vi "SVFA Get Spectrum Value (NxM).vi"(0 "spectra":T8(array[cluster]) {"magnitude" format="%.2f"; "dx" format="%.2f"; "x0" format="%.2f"}, 2 "x value (1000)":dbl=1000.0 format="%.2f", 3 "coercion (nearest)":T1(ring), 4 "spectrum info":T2[][](array[typedef]) {"x-axis units" items=["Frequency-Arbitrary (Hz)"=0, "Frequency-CB (Hz)"=1, "Frequency-CPB (Hz)"=1248, "Frequency-Arbitrary (Hz)"=2357, "Quefrency (s)"=2, "Revolutions (rev)"=3, "Order"=4, "Speed (RPM)"=11, "Speed (rad/s)"=21, "Index"=65535]; "weighting filter" items=["Linear", "A-weighting", "B-weighting", "C-weighting", "ITU-R 468-4", "Dolby", "CCITT", "C-message", "Wb", "Wc", "Wd", "We", "Wf", "Wh", "Wj", "Wk", "Wm", "AES17 20 kHz lowpass", "AES17 40 kHz lowpass", "AES17 20 kHz highpass", "AES17 40 kHz highpass"]; "dB reference [EU]" format="%.2f"; "engineering units" items=["custom..."=0, "V"=1, "A"=21, "C"=30, "pC"=31, "s"=32, "-"=29, "Pa"=2, "N"=20, "g"=3, "m/s^2"=4, "m/s"=5, "m"=6, "mm/s"=12, "mm"=13, "micron/s"=14, "micron"=15, "in/s^2"=7, "in/s"=8, "in"=9, "mil/s"=10, "mil"=11, "rad/s^2"=16, "rad/s"=17, "rad"=18, "deg/s^2"=26, "deg/s"=27, "deg"=28, "RPM"=22, "cycle/s^2"=23, "Hz"=24, "cycle"=25, "strain"=19]; "spectral info"."window" items=["None "=0, "Hanning"=1, "Hamming"=2, "Blackman-Harris"=3, "Exact Blackman"=4, "Blackman"=5, "Flat Top"=6, "4 Term B-Harris "=7, "7 Term B-Harris"=8, "Low Sidelobe"=9, "Force - Exponential"=10, "Gaussian"=62]}, 5 "error in (no error)":errorcluster) -> (14 "spectra values":dbl[][](array[numeric]), 15 "unit labels":string[][](array[string]), 16 "actual x values":dbl[][](array[numeric]), 17 "x labels":string[][](array[string]), 19 "error out":errorcluster)   [LabVIEW 2017]
doc: "Extracts the value of the spectrum at the specified frequency. Use the frequency coercion control to specify how the frequency should be coerced if it does not exactly coincide with a frequency line. This VI operates on any real-valued spectrum. Wire data to the <B>spectrum</B> input to determine the polymorphic instance to use or manually select the instance."
uses:
  <vilib>/addons/_NISVFA/_Shared subVIs/Controls/svc_Spectrum Info.ctl
  <vilib>/addons/_NISVFA/_Shared subVIs/Controls/svc_X-Axis Units.ctl
  <vilib>/addons/_NISVFA/_Shared subVIs/Controls/svc_Spectrum Type.ctl
  <vilib>/addons/_NISVFA/_Shared subVIs/Controls/svc_Engineering Units Text Ring.ctl
  <vilib>/addons/_NISVFA/_Shared subVIs/Controls/svc_Weighting Filter Text Ring.ctl
  <vilib>/addons/_NISVFA/_Shared subVIs/Controls/svc_Complimentary Spectrum Units.ctl
  <vilib>/addons/_NISVFA/_Shared subVIs/Common/svc_Spectrum Units.vi
  <vilib>/addons/_NISVFA/_Shared subVIs/Common/svc_Convert Frequency to Frequency String.vi
  <vilib>/addons/_NISVFA/_Shared subVIs/Common/svc_Get Weighting Enum and Labels.vi
  <vilib>/addons/_NISVFA/_Shared subVIs/Common/svc_Unit Label Lexical Class.vi
  <vilib>/addons/_NISVFA/_Shared subVIs/Common/svc_Engineering Units to Unit Label.vi
  <vilib>/addons/_NISVFA/_Shared subVIs/Common/svc_Format Value (DBL).vi
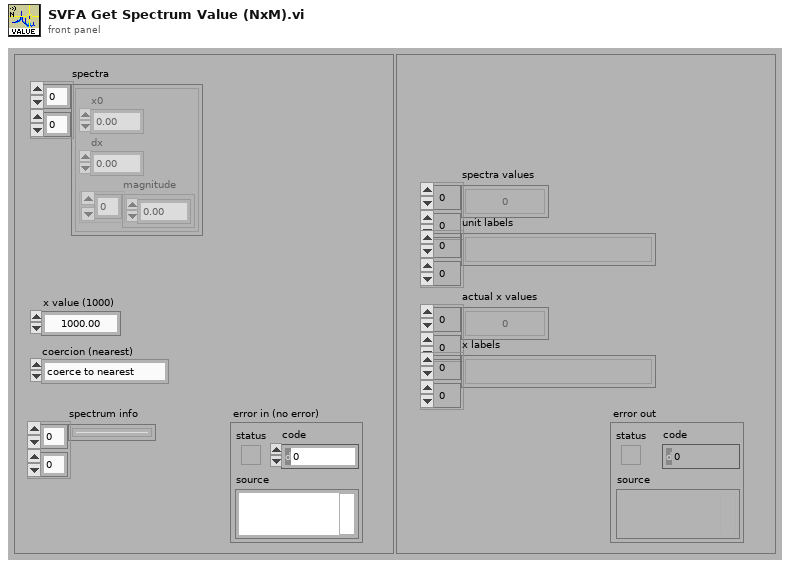
[diagram p1: front panel]
types:
  T1 = enum16{"coerce to nearest", "coerce to next highest", "coerce to next lowest", "interpolate"}
  T2 = typedef "svc_Spectrum Info.ctl" = cluster{"channel name":string, "description":string, "x-axis units":T3, "spectral info":cluster{"spectrum type":T4, "linear/dB":enum16{"linear", "dB"}, "window":u16, "window size":i32, "FFT size":i32}, "engineering units":T5, "custom label":string, "dB reference [EU]":dbl, "peak units":enum16{"rms", "peak", "peak-peak"}, "weighting filter":T6, "spectral density?":bool, "unit label":string, "spectrum skewed?":bool, "complimentary spectrum units":T7}
  T3 = typedef "svc_X-Axis Units.ctl" = u16
  T4 = typedef "svc_Spectrum Type.ctl" = enum16{"FFT Spectrum [complex]", "Amplitude [Magnitude]", "Power [Magnitude^2]", "Cross Spectrum [complex]", "Frequency Response [Complex]"}
  T5 = typedef "svc_Engineering Units Text Ring.ctl" = u16
  T6 = typedef "svc_Weighting Filter Text Ring.ctl" = u16
  T7 = typedef "svc_Complimentary Spectrum Units.ctl" = enum16{"none", "radians", "degrees", "cycles", "imaginary"}
  T8 = cluster{"x0":dbl, "dx":dbl, "magnitude":dbl[]}[][]
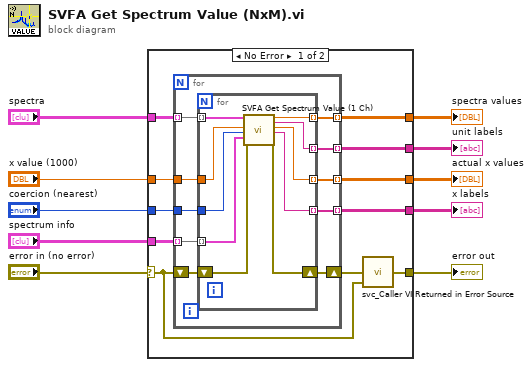
[diagram p0: block diagram]
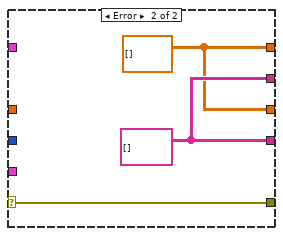
[diagram p2: hidden frame]
diagram:
  n1 = case shown="No Error" "error in (no error)" {
    tunnel: [w20 w44] -> w10
    tunnel: "spectrum info" -> [w18 _]
    tunnel: "spectra" -> [w19 _]
    tunnel: [w17 w42] -> w7
    tunnel: [w16 w43] -> w4
    tunnel: "x value (1000)" -> [w15 _]
    tunnel: "coercion (nearest)" -> [w14 _]
    tunnel: [w13 w42] -> w3
    selector: "error in (no error)" -> [w11 w44]
    tunnel: [w12 w43] -> w2
    frame No Error {
      n2 = for {
        tunnel: w19 -> [w29] mode=indexing
        tunnel: w18 -> [w28] mode=indexing
        tunnel: [w27] -> w17 mode=indexing
        tunnel: [w26] -> w16 mode=indexing
        tunnel: w15 -> [w22]
        tunnel: w14 -> [w23]
        tunnel: [w25] -> w13 mode=indexing
        shift-right: [w30] -> w21
        shift-left: w11 -> [w31]
        tunnel: [w24] -> w12 mode=indexing
        n3 = for {
          tunnel: w29 -> [w39] mode=indexing
          tunnel: w28 -> [w38] mode=indexing
          tunnel: [w37] -> w27 mode=indexing
          tunnel: [w36] -> w26 mode=indexing
          tunnel: [w35] -> w25 mode=indexing
          tunnel: [w34] -> w24 mode=indexing
          tunnel: w23 -> [w33]
          tunnel: w22 -> [w32]
          shift-right: [w40] -> w30
          shift-left: w31 -> [w41]
          n4 = call <vilib>:"SVFA Get Spectrum Value (1 Ch).vi"("spectrum"=w39, "x value (1000)"=w32, "coercion (nearest)"=w33, "spectrum info"=w38, "error in (no error)"=w41) -> ("spectrum value"=w37:dbl, "unit label"=w36:string, "actual x value"=w35:dbl, "x label"=w34:string, "error out"=w40:errorcluster)  [unwired: 10 in]
        }
      }
      n5 = call <vilib>:"svc_Caller VI Returned in Error Source.vi"("warning input to caller"=w11, "error in (no error)"=w21) -> ("error out"=w20:errorcluster)  [unwired: 3 in]
    }
    frame Error {
      w43 = string[][] []
      w42 = dbl[][] [] ("Array")
    }
  }
  "error out" <- w10
  "spectra values" <- w7
  "actual x values" <- w3
  "unit labels" <- w4
  "x labels" <- w2
